vi "test Get Firmware Version.vi"(11 "Test Case In":refnum<class "Test PCANBasic.lvclass">) -> (0 "error out":errorcluster, 3 "Test Case Out":refnum<class "Test PCANBasic.lvclass">)   [LabVIEW 2020, in "Test PCANBasic.lvclass"]
uses:
  Test PCANBasic.lvclass
  C:/Program Files/National Instruments/LabVIEW 2025/vi.lib/Astemes/LUnit/Test Case.lvclass
  <vilib>/Astemes/LUnit/Test Case.lvclass/Test Case.ctl
  Test PCANBasic.lvclass/Test PCANBasic.ctl
  source/PCANBasic.lvlib
  <vilib>/Astemes/LUnit/Test Case.lvclass
  Global PCAN Channel.vi
  Global PCAN Baudrate.vi
panel:
  out "Firmware Version":string
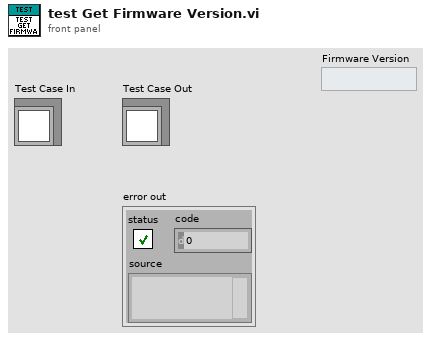
[diagram p1: front panel]
types:
  T1 = typedef "PCANBasic.lvlib/TPCANHandle.ctl" = u16
  T2 = typedef "PCANBasic.lvlib/PCAN Baud.ctl" = u16
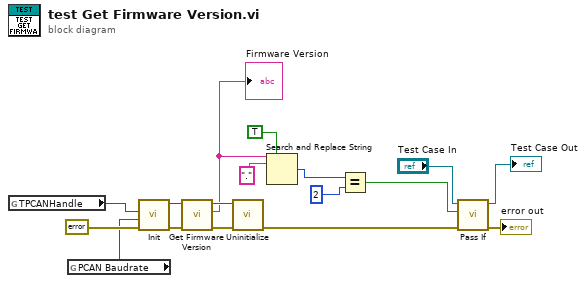
[diagram p0: block diagram]
diagram:
  n1 = global read "Global PCAN Channel.vi" "TPCANHandle"() -> (w2:T1)
  n2 = global read "Global PCAN Baudrate.vi" "PCAN Baudrate"() -> (w10:T2)
  n3 = call "Init.vi"("error in"=errorcluster {"status"=FALSE, "code"=0, "source"=""}, "Baudrate"=w10, "Channel"=w2) -> ("error out"=w12:errorcluster, "TPCANHandle out"=w11:T1)  [unwired: 6 in, 1 out]
  n4 = call "Get Firmware Version.vi"("error in"=w12, "TPCANHandle in"=w11) -> ("error out"=w14:errorcluster, "Firmware Version"=w1:string, "TPCANHandle out"=w8:T1)  [unwired: 6 in, 1 out]
  "Firmware Version" <- w1
  n5 = call "Uninitialize.vi"("error in"=w14, "TPCANHandle in"=w8) -> ("error out"=w9:errorcluster)  [unwired: 8 in, 1 out]
  n6 = Search and Replace String(replace all?=TRUE ("replace all? (F)"), input string=w1, search string=".") -> (number of replacements=w5:i32)  [unwired: 5 in, 3 out]
  n7 = Equal?(x=w5, y=2) -> (x = y?=w3:bool)
  n8 = call <vilib>:"Pass If.vi"("error in (no error)"=w9, "Pass?"=w3, "LUnit Test Case In"="Test Case In") -> ("error out"=→"error out":errorcluster, "LUnit Test Case Out"=→"Test Case Out":refnum<class "Test PCANBasic.lvclass">)  [unwired: 7 in]
